vi "Update Subsystem Alarm Status.vi"(8 "error in (no error)":errorcluster, 10 "Subsystem URL":refnum<k21>, 11 "Reference URL Map In":variant) -> (0 "error out":errorcluster, 3 "Reference URL Map Out":variant)   [LabVIEW 2024]
doc: "Updates the alarm status for a subsystem."
uses:
  <vilib>/lvdsc/NI_DSC.lvlib
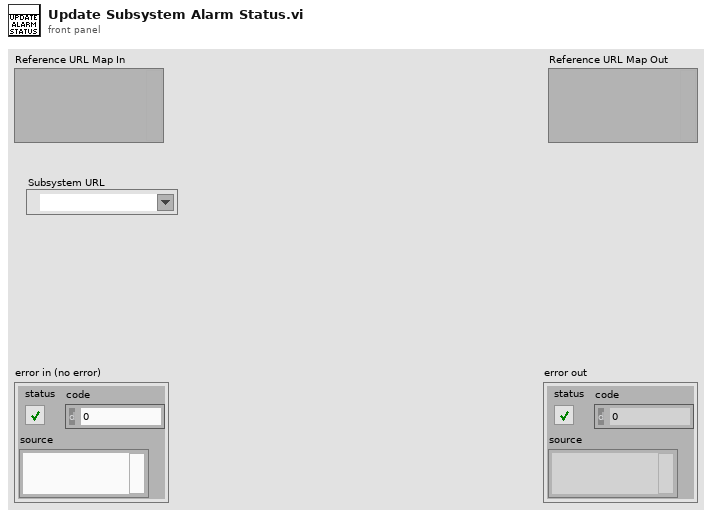
[diagram p1: front panel]
types:
  T1 = cluster{"Min priority":u32, "Max priority":u32, "Show Acknowledged alarms?":bool}
  T2 = cluster{"# active alarms occurrences":i32, "any alarm occurrences?":bool, "# unack alarms occurrences":i32, "any unack alarm occurrences?":bool, "# shared variables with active alarms":i32, "any shared variables with alarms?":bool, "# shared variables with unack alarms":i32, "any shared variables with unack alarms?":bool}
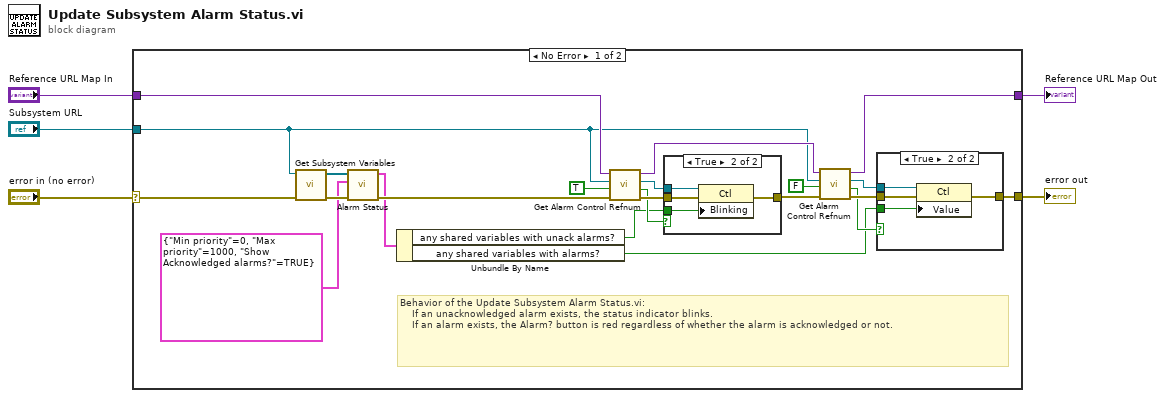
[diagram p0: block diagram]
diagram:
  n1 = case shown="No Error" "error in (no error)" {
    selector: "error in (no error)" -> [w12 w39]
    tunnel: [w18 w39] -> w4
    tunnel: "Reference URL Map In" -> [w27 w38]
    tunnel: [w26 w38] -> w2
    tunnel: "Subsystem URL" -> [w13 _]
    frame No Error {
      # "Behavior of the Update Subsystem Alarm Status.vi:\n    If an unacknowledged alarm exists, the status indicator blinks.\n    If an alarm exists, the Alarm? button is red regardless of whether the alarm is acknowledged or not."
      n2 = call "Get Subsystem Variables.vi"("error in (no error)"=w12, "Subsystem URL"=w13) -> ("error out"=w11:errorcluster, "Variable URLs"=w10:refnum<k21>[])  [unwired: 6 in, 2 out]
      n3 = call <vilib>:"Alarm Status.vi"("error in (no error)"=w11, "read parameters"=T1 {"Min priority"=0, "Max priority"=1000, "Show Acknowledged alarms?"=TRUE}, "shared variables"=w10) -> ("error out"=w17:errorcluster, "alarm summary data"=w9:T2)  [unwired: 7 in]
      n4 = Unbundle By Name(w9) -> ("any shared variables with unack alarms?"=w7:bool, "any shared variables with alarms?"=w6:bool)
      n5 = call "Get Alarm Control Refnum.vi"("error in (no error)"=w17, "Active Alarm?"=TRUE, "Subsystem URL"=w13, "Reference URL Map In"=w27) -> ("error out"=w23:errorcluster, "Found?"=w22:bool, "Control Refnum"=w16:refnum<vi>, "Reference URL Map Out"=w21:variant)  [unwired: 4 in]
      n6 = case shown="True" w22 {
        tunnel: [w28 w32] -> w24
        tunnel: w7 -> [_ w31]
        tunnel: w23 -> [w28 w30]
        tunnel: w16 -> [_ w29]
        frame False {
        }
        frame True {
          n7 = property class="Ctl"(reference=w29, error in=w30, "Blinking"=w31) -> (error out=w32:errorcluster)  [unwired: 1 out]
        }
      }
      n8 = call "Get Alarm Control Refnum.vi"("error in (no error)"=w24, "Active Alarm?"=FALSE, "Subsystem URL"=w13, "Reference URL Map In"=w21) -> ("error out"=w25:errorcluster, "Found?"=w20:bool, "Control Refnum"=w19:refnum<vi>, "Reference URL Map Out"=w26:variant)  [unwired: 4 in]
      n9 = case shown="True" w20 {
        tunnel: [w33 w37] -> w18
        tunnel: w6 -> [_ w36]
        tunnel: w25 -> [w33 w35]
        tunnel: w19 -> [_ w34]
        frame False {
        }
        frame True {
          n10 = property class="Ctl"(reference=w34, error in=w35, "Value"=w36) -> (error out=w37:errorcluster)  [unwired: 1 out]
        }
      }
    }
    frame Error {
    }
  }
  "error out" <- w4
  "Reference URL Map Out" <- w2
